vi "runrate.vi"   [LabVIEW 2012]
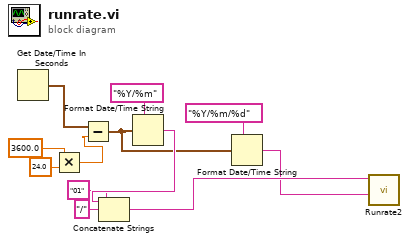
[diagram p0: block diagram]
diagram:
  n1 = Get Date/Time In Seconds() -> (seconds since 1Jan1904=w12:timestamp)
  n2 = Multiply(x=3600.0, y=24.0) -> (x*y=w10:dbl)
  n3 = Subtract(x=w12, y=w10) -> (x-y=w3:timestamp)
  n4 = Format Date/Time String(time format string (%c)="%Y/%m", seconds (now)=w3) -> (date/time string=w6:string)  [unwired: 1 in]
  n5 = Concatenate Strings(w6, "/" ("string"), "01" ("string")) -> (w2:string)
  n6 = Format Date/Time String(time format string (%c)="%Y/%m/%d", seconds (now)=w3) -> (date/time string=w1:string)  [unwired: 1 in]
  n7 = call "Runrate2.vi"("EndDate"=w1, "BegDate"=w2) -> ()  [unwired: 10 in]
